vi "GetProperties.vi"(8 "error in":errorcluster, 11 "RotaryColorScale in":refnum<class "RotaryColorScale.lvclass">) -> (0 "error out":errorcluster, 3 "RotaryColorScale out":refnum<class "RotaryColorScale.lvclass">)   [LabVIEW 2014, in "Raspberry Pi Compatible Compiler for LabVIEW.lvlib" / "RotaryColorScale.lvclass"]
uses:
  RotaryColorScale.lvclass
  RotaryColorScale.lvclass/RotaryColorScale.ctl
  ColorScale/ColorScale.lvclass
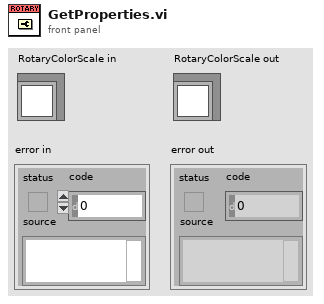
[diagram p1: front panel]
types:
  T1 = typedef "LVScalePositionTypeDef.ctl" = cluster{"Start":dbl, "Range":dbl}
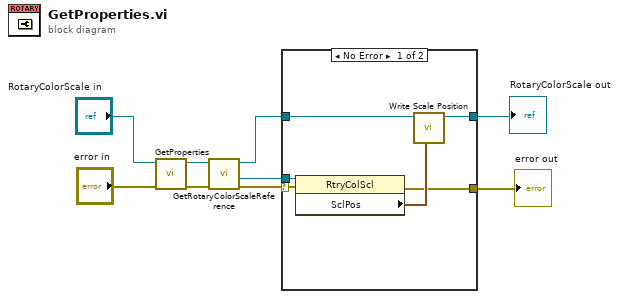
[diagram p0: block diagram]
diagram:
  n1 = call-parent "GetProperties.vi"("error in"="error in", "ColorScale in"="RotaryColorScale in") -> ("error out"=w6:errorcluster, "ColorScale out"=w7:refnum<class "RotaryColorScale.lvclass">)  [unwired: 8 in]
  n2 = call "GetRotaryColorScaleReference.vi"("error in"=w6, "RotaryColorScale in"=w7) -> ("error out"=w5:errorcluster, "color scale reference"=w4:refnum<vi>, "RotaryColorScale out"=w3:refnum<class "RotaryColorScale.lvclass">)  [unwired: 7 in]
  n3 = case shown="No Error" w5 {
    selector: w5 -> [w15 w16]
    tunnel: w4 -> [w14 _]
    tunnel: w3 -> [w13 w17]
    tunnel: [w11 w17] -> w2
    tunnel: [w10 w16] -> w1
    frame No Error {
      n4 = property class="RtryColScl"(reference=w14, error in=w15) -> (error out=w10:errorcluster, "SclPos"=w12:T1)  [unwired: 1 out]
      n5 = call "Write Scale Position.vi"("Scale Position"=w12, "RotaryColorScale in"=w13) -> ("RotaryColorScale out"=w11:refnum<class "RotaryColorScale.lvclass">)  [unwired: 7 in]
    }
    frame Error {
    }
  }
  "error out" <- w1
  "RotaryColorScale out" <- w2
